vi "JoystickToDial Demo.vi"(7 "Reset":bool, 9 "Reverse":bool, 10 "Y":dbl, 11 "X":dbl) -> (3 "Heading":dbl(knob) scale=-360.0..360.0)   [LabVIEW 2016]
uses:
  <vilib>/Rock Robotics/Network Tables/NT Read Numeric Array.vi
  <vilib>/Rock Robotics/Network Tables/NT Read Boolean.vi
  <vilib>/Rock Robotics/Network Tables/NT Write Number.vi
  <vilib>/Rock Robotics/Network Tables/NT Write Numeric Array.vi
panel:
  out "Meter":dbl(knob) scale=-1.0..1.0
  in  "Leave this false":bool
  out "Y":dbl
  out "X":dbl
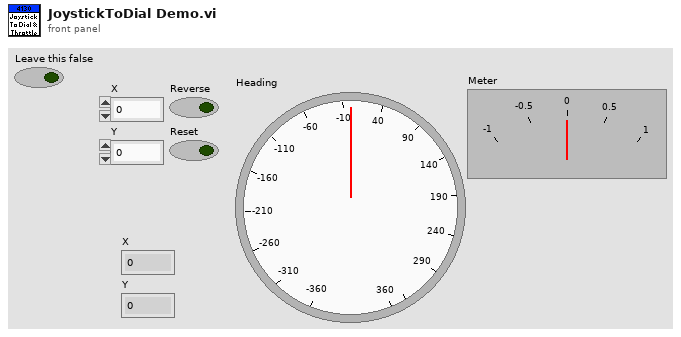
[diagram p1: front panel]
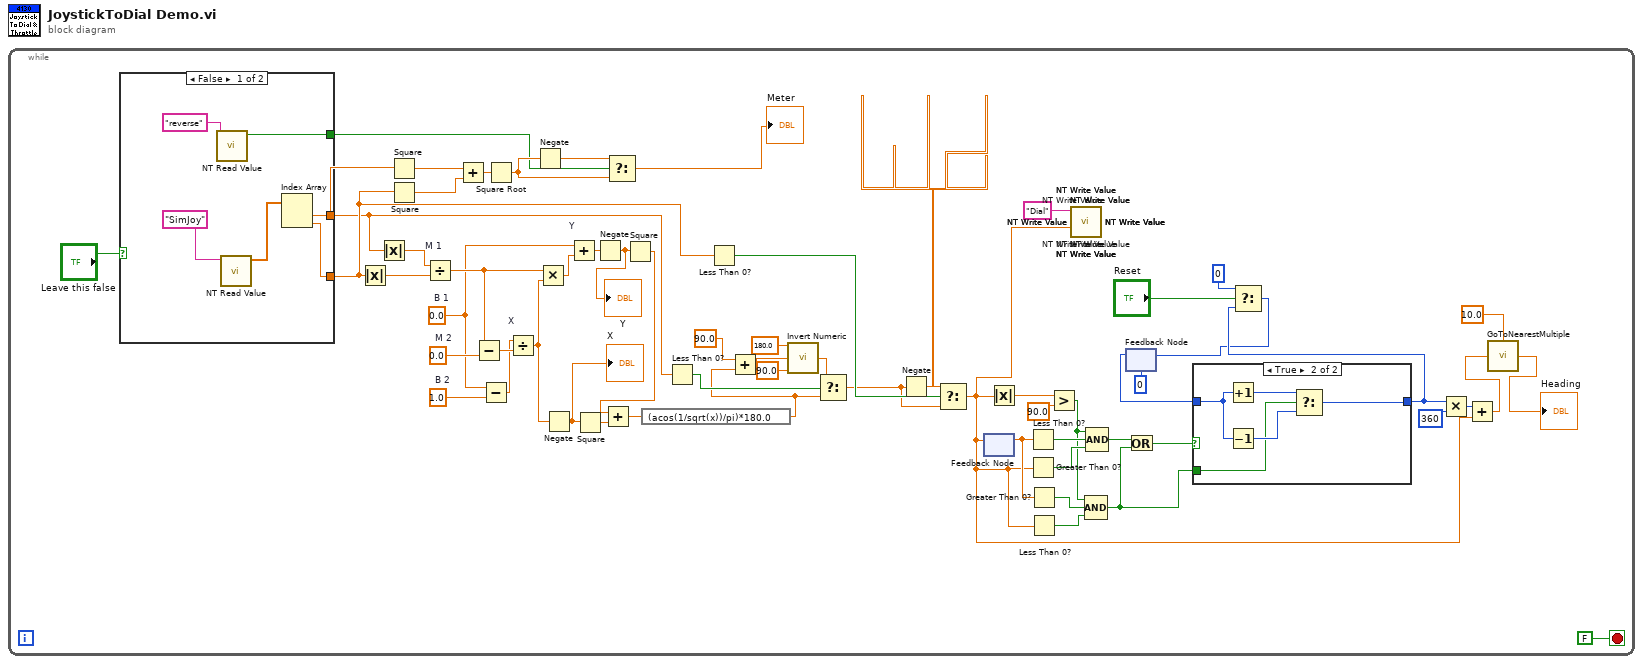
[diagram p0: block diagram]
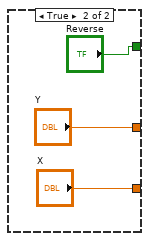
[diagram p2: hidden frame]
diagram:
  n1 = while {
    stop <- FALSE stop-if-true
    w60 = 0.0  # M 2
    w61 = 1.0  # B 2
    w49 = 0.0  # B 1
    n2 = case shown="False" "Leave this false" {
      tunnel: [w64 "X"] -> w17
      tunnel: [w65 "Y"] -> w16
      tunnel: [w63 "Reverse"] -> w6
      frame False {
        n3 = call-poly <vilib>:"NT Read Value.vi"("Name"="reverse") -> ("Boolean"=w63:bool)  [unwired: 9 in, 1 out]
        n4 = call-poly <vilib>:"NT Read Value.vi"("Name"="SimJoy") -> ("Numeric Array"=w66:dbl[])  [unwired: 9 in, 1 out]
        n5 = Index Array(array=w66) -> (element #1=w65:dbl, element #2=w64:dbl)  [unwired: 2 in]
      }
      frame True {
      }
    }
    n6 = Absolute Value(x=w17) -> (abs(x)=w50:dbl)
    n7 = Absolute Value(x=w16) -> (abs(x)=w51:dbl)
    n8 = Square(x=w16) -> (x^2=w22:dbl)
    n9 = Square(x=w17) -> (x^2=w21:dbl)
    n10 = Divide "M 1"(x=w51, y=w50) -> (x/y=w59:dbl)
    n11 = Add(x=w22, y=w21) -> (x+y=w20:dbl)
    n12 = Subtract(x=w59, y=w60) -> (x-y=w57:dbl)
    n13 = Subtract(x=w49, y=w61) -> (x-y=w56:dbl)
    n14 = Square Root(x=w20) -> (sqrt(x)=w19:dbl)
    n15 = Divide "X"(x=w56, y=w57) -> (x/y=w38:dbl)
    n16 = Negate(x=w19) -> (-x=w4:dbl)
    n17 = Multiply(x=w59, y=w38) -> (x*y=w58:dbl)
    n18 = Negate(x=w38) -> (-x=w55:dbl)
    "X" <- w55
    n19 = Add "Y"(x=w49, y=w58) -> (x+y=w18:dbl)
    n20 = Square(x=w55) -> (x^2=w53:dbl)
    n21 = Negate(x=w18) -> (-x=w11:dbl)
    "Y" <- w11
    n22 = Select(t=w4, s=w6, f=w19) -> (s? t:f=→"Meter":dbl)
    n23 = Square(x=w11) -> (x^2=w54:dbl)
    n24 = Add(x=w54, y=w53) -> (x+y=w52:dbl)
    n25 = expression code="(acos(1/sqrt(x))/pi)*180.0"(w52) -> (w45:dbl)
    n26 = Less Than 0?(x=w16) -> (x < 0?=w48:bool)
    n27 = Less Than 0?(x=w17) -> (x < 0?=w46:bool)
    n28 = Add(x=90.0, y=w45) -> (x+y=w42:dbl)
    n29 = call "Invert Numeric.vi"("celing"=180.0, "Numeric"=w42, "floor"=90.0) -> ("Inverted"=w41:dbl)  [unwired: 10 in, 2 out]
    n30 = Select(t=w41, s=w48, f=w45) -> (s? t:f=w40:dbl)
    n31 = Negate(x=w40) -> (-x=w39:dbl)
    n32 = Select(t=w39, s=w46, f=w40) -> (s? t:f=w7:dbl)
    n33 = feedback #1() -> (w29:dbl)  [unwired: 1 in]
    n34 = feedback-in #1(w7) -> ()
    n35 = Absolute Value(x=w7) -> (abs(x)=w32:dbl)
    n36 = Less Than 0?(x=w29) -> (x < 0?=w31:bool)
    n37 = Greater Than 0?(x=w7) -> (x > 0?=w30:bool)
    n38 = Greater Than 0?(x=w29) -> (x > 0?=w27:bool)
    n39 = Less Than 0?(x=w7) -> (x < 0?=w26:bool)
    n40 = Greater?(x=w32, y=90.0) -> (0:w28:bool)
    n41 = call-poly <vilib>:"NT Write Value.vi"("Numeric"=w7, "Name"="Dial") -> ()  [unwired: 9 in, 1 out]
    n42 = call-poly <vilib>:"NT Write Value.vi"() -> ()  [unwired: 11 in, 1 out]
    n43 = call-poly <vilib>:"NT Write Value.vi"() -> ()  [unwired: 11 in, 1 out]
    n44 = call-poly <vilib>:"NT Write Value.vi"() -> ()  [unwired: 11 in, 1 out]
    n45 = call-poly <vilib>:"NT Write Value.vi"() -> ()  [unwired: 11 in, 1 out]
    n46 = call-poly <vilib>:"NT Write Value.vi"() -> ()  [unwired: 11 in, 1 out]
    n47 = call-poly <vilib>:"NT Write Value.vi"() -> ()  [unwired: 11 in, 1 out]
    n48 = call-poly <vilib>:"NT Write Value.vi"() -> ()  [unwired: 11 in, 1 out]
    n49 = call-poly <vilib>:"NT Write Value.vi"() -> ()  [unwired: 11 in, 1 out]
    n50 = call-poly <vilib>:"NT Write Value.vi"() -> ()  [unwired: 11 in, 1 out]
    n51 = call-poly <vilib>:"NT Write Value.vi"() -> ()  [unwired: 11 in, 1 out]
    n52 = call-poly <vilib>:"NT Write Value.vi"() -> ()  [unwired: 11 in, 1 out]
    n53 = call-poly <vilib>:"NT Write Value.vi"() -> ()  [unwired: 11 in, 1 out]
    n54 = call-poly <vilib>:"NT Write Value.vi"() -> ()  [unwired: 11 in, 1 out]
    n55 = call-poly <vilib>:"NT Write Value.vi"() -> ()  [unwired: 11 in, 1 out]
    n56 = call-poly <vilib>:"NT Write Value.vi"() -> ()  [unwired: 11 in, 1 out]
    n57 = Compound Arithmetic op=AND(w28, w27, w26) -> (w23:bool)
    n58 = Compound Arithmetic op=AND(w28, w31, w30) -> (w24:bool)
    n59 = feedback #2(0) -> (w37:i32)
    n60 = Or(x=w24, y=w23) -> (x .or. y?=w25:bool)
    n61 = case shown="True" w25 {
      tunnel: [w71 w74] -> w15
      tunnel: w37 -> [w71 w73]
      tunnel: w23 -> [_ w72]
      frame False {
      }
      frame True {
        n62 = Increment(x=w73) -> (x+1=w75:i32)
        n63 = Decrement(x=w73) -> (x-1=w76:i32)
        n64 = Select(t=w75, s=w72, f=w76) -> (s? t:f=w74:i32)
      }
    }
    n65 = Select(t=0, s="Reset", f=w15) -> (s? t:f=w14:i32)
    n66 = feedback-in #2(w14) -> ()
    n67 = Multiply(x=w15, y=360) -> (x*y=w34:i32)
    n68 = Add(x=w34, y=w7) -> (x+y=w3:dbl)
    n69 = call "GoToNearestMultiple.vi"("Multiple"=10.0, "Numeric"=w3) -> ("Numeric"=→"Heading":dbl)  [unwired: 13 in]
  }
